vi "lacz_nazwe_z_cyfra.vi"(6 "num i":i32, 9 "name in":string) -> (5 "name out":string)   [LabVIEW 2014]
doc: "Łączy nazwę i cyfrę wejściową w jeden ciąg znaków string"
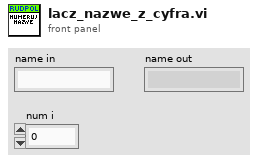
[diagram p1: front panel]
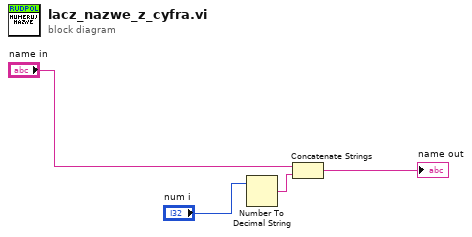
[diagram p0: block diagram]
diagram:
  n1 = Number To Decimal String(number="num i") -> (decimal integer string=w2:string)  [unwired: 1 in]
  n2 = Concatenate Strings("name in", w2) -> (→"name out":string)
